vi "Read Connection Settings.vi"(8 "error in (no error)":errorcluster, 11 "Boot Loader in":refnum<class "Boot Loader.lvclass">) -> (0 "error out":errorcluster, 2 "Connection Settings":T1={"Pressure Servo Valve 1 DAC"=1, "Pressure Servo Valve 2 DAC"=2, "Turbo Valve DAC"=3, "Load Cell ADC"=1, "FC1 ILC Port"="", "FC2 ILC Port"="", "Tovey A-B Port"="", "Tovey C-F Port"="", "Tovey D-E Port"="", "FC1 ILC Protocol"=enum."RS485", "FC2 ILC Protocol"=enum."RS485", "Tovey A-B Protocol"=enum."RS485", "Tovey C-F Protocol"=enum."RS485", "Tovey D-E Protocol"=enum."RS485", "Tovey A-B Address"=3, "Tovey C-F Address"=1, "Tovey D-E Address"=1} {"Tovey D-E Address" min=1; "Tovey C-F Address" min=1; "Tovey A-B Address" min=1; "Load Cell ADC" min=1 max=4; "Turbo Valve DAC" min=1 max=4; "Pressure Servo Valve 2 DAC" min=1 max=4; "Pressure Servo Valve 1 DAC" min=1 max=4}, 3 "Boot Loader out":refnum<class "Boot Loader.lvclass">)   [LabVIEW 2015, in "Boot Loader.lvclass"]
uses:
  Boot Loader.lvclass
  Typedefs/Connection Settings.ctl
  <userlib>/Common/SerialProtocols/Configuration/SerialProtocol.ctl
  Settings/Settings.lvclass
  <userlib>/Common/SerialProtocols/SerialProtocols.lvlib
  Typedefs/FAMT Typedefs.lvlib
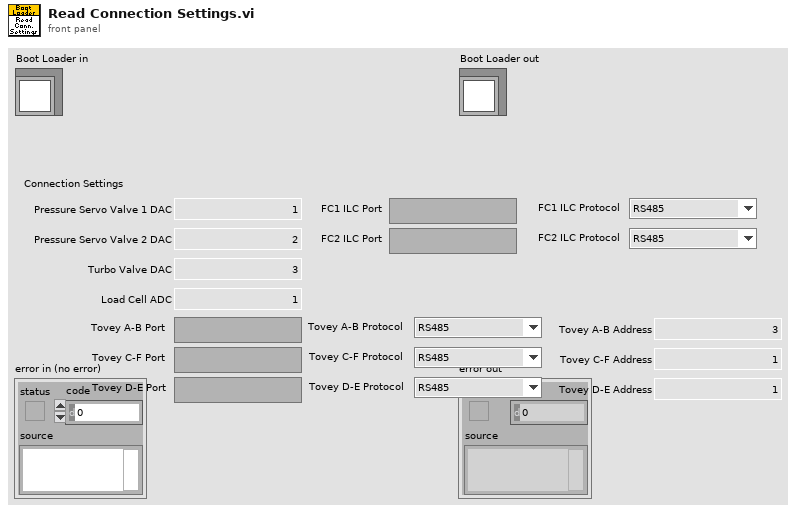
[diagram p1: front panel]
types:
  T1 = typedef "FAMT Typedefs.lvlib/Connection Settings.ctl" = cluster{"Pressure Servo Valve 1 DAC":u8, "Pressure Servo Valve 2 DAC":u8, "Turbo Valve DAC":u8, "Load Cell ADC":u8, "FC1 ILC Port":refnum<visa-resource-name>, "FC2 ILC Port":refnum<visa-resource-name>, "Tovey A-B Port":refnum<visa-resource-name>, "Tovey C-F Port":refnum<visa-resource-name>, "Tovey D-E Port":refnum<visa-resource-name>, "FC1 ILC Protocol":T2, "FC2 ILC Protocol":T2, "Tovey A-B Protocol":T2, "Tovey C-F Protocol":T2, "Tovey D-E Protocol":T2, "Tovey A-B Address":u8, "Tovey C-F Address":u8, "Tovey D-E Address":u8}
  T2 = typedef "SerialProtocols.lvlib/SerialProtocol.ctl" = enum16{"RS232", "RS485", "SerialSimulator"}
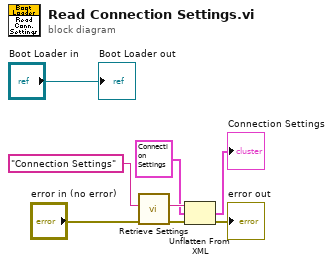
[diagram p0: block diagram]
diagram:
  n1 = call "Retrieve Settings.vi"("error in (no error)"="error in (no error)", "configName"="Connection Settings") -> ("error out"=w4:errorcluster, "xmlConfig"=w7:string)  [unwired: 7 in, 1 out]
  n2 = Unflatten From XML(xml string=w7, type=T1 {"Pressure Servo Valve 1 DAC"=1, "Pressure Servo Valve 2 DAC"=2, "Turbo Valve DAC"=3, "Load Cell ADC"=1, "FC1 ILC Port"="", "FC2 ILC Port"="", "Tovey A-B Port"="", "Tovey C-F Port"="", "Tovey D-E Port"="", "FC1 ILC Protocol"=enum."RS485", "FC2 ILC Protocol"=enum."RS485", "Tovey A-B Protocol"=enum."RS485", "Tovey C-F Protocol"=enum."RS485", "Tovey D-E Protocol"=enum."RS485", "Tovey A-B Address"=3, "Tovey C-F Address"=1, "Tovey D-E Address"=1} ("Connection Settings"), error in (no error)=w4) -> (value=→"Connection Settings":T1, error out=→"error out":errorcluster)
  "Boot Loader out" <- "Boot Loader in"
